vi "Perform Search Packages.vi"(9 "Filters":T1, 10 "SearchCriteria":string, 11 "All Packages":refnum<class "Package.lvclass">[](array[class])) -> (3 "Found Packages":refnum<class "Package.lvclass">[](array[class]))   [LabVIEW 2020, in "WSsupport.lvlib"]
uses:
  WSsupport.lvlib
  Packages/Package_class/Package.lvclass
  Packages/Package Version_class/Package Version.lvclass
  Search Filters.ctl
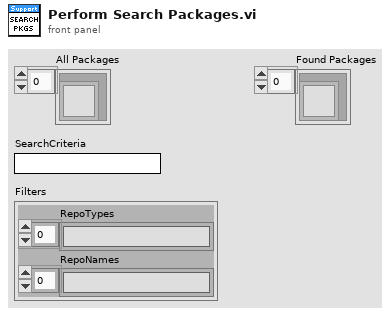
[diagram p1: front panel]
types:
  T1 = typedef "WSsupport.lvlib/Search Filters.ctl" = cluster{"RepoTypes":string[], "RepoNames":string[]}
  T2 = typedef "Packages.lvlib/Repo.lvclass/RepoType--enum.ctl" = enum16{"VIPM", "NIPM", "GPM"}
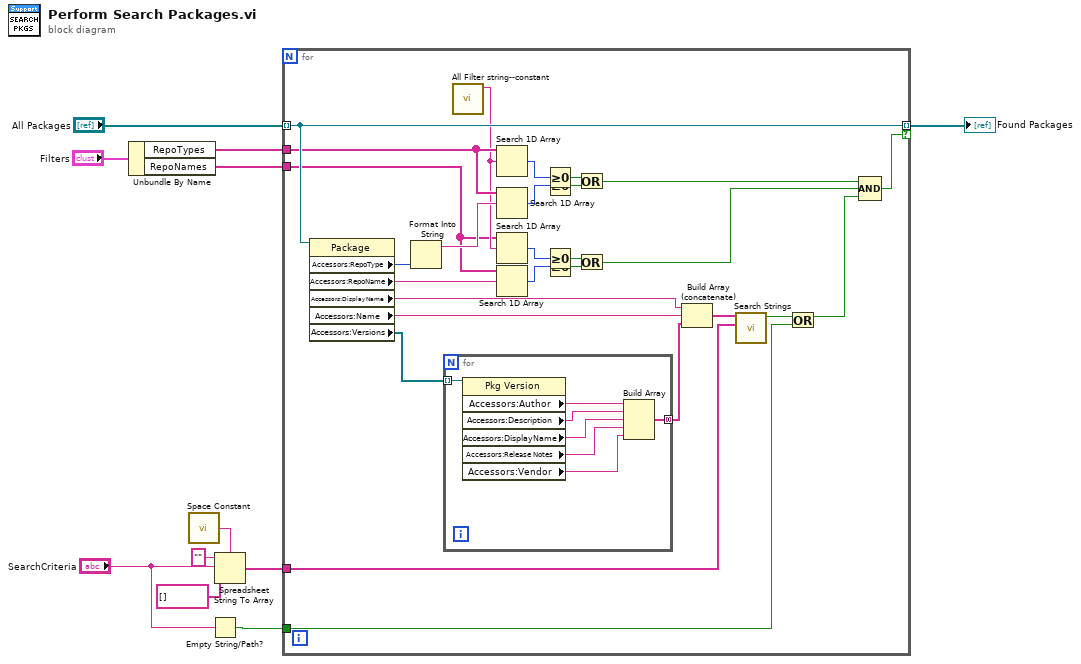
[diagram p0: block diagram]
diagram:
  n1 = Unbundle By Name("Filters") -> ("RepoTypes"=w2:string[], "RepoNames"=w1:string[])
  n2 = call <vilib>:"Space Constant.vi"() -> ("String"=w7:string)
  n3 = Empty String/Path?(string/path="SearchCriteria") -> (empty?=w4:bool)
  n4 = Spreadsheet String To Array(delimiter (Tab)=w7, format string="", spreadsheet string="SearchCriteria", array type (2D Dbl)=string[] []) -> (array=w5:string[])
  n5 = for {
    tunnel: "All Packages" -> [w37] mode=indexing
    tunnel: w5 -> [w32]
    tunnel: [w37] -> w10 mode=indexing if=w27
    tunnel: w4 -> [w29]
    tunnel: w2 -> [w26]
    tunnel: w1 -> [w19]
    n6 = property class="Package"(reference=w37) -> ("Accessors:RepoType"=w28:T2, "Accessors:RepoName"=w20:string, "Accessors:DisplayName"=w35:string, "Accessors:Name"=w34:string, "Accessors:Versions"=w38:refnum<class "Package Version.lvclass">[])  [unwired: 1 in, 2 out]
    n7 = Format Into String(w28) -> (resulting string=w25:string)  [unwired: 3 in, 1 out]
    n8 = for {
      tunnel: w38 -> [w45] mode=indexing
      tunnel: [w39] -> w36 mode=concatenating
      n9 = property class="Pkg Version"(reference=w45) -> ("Accessors:Author"=w44:string, "Accessors:Description"=w43:string, "Accessors:DisplayName"=w42:string, "Accessors:Release Notes"=w41:string, "Accessors:Vendor"=w40:string)  [unwired: 1 in, 2 out]
      n10 = Build Array(w44, w43, w42, w41, w40) -> (w39:string[])
    }
    n11 = call "All Filter string--constant.vi"() -> ("All Filter string"=w21:string)  [unwired: 11 in]
    n12 = Search 1D Array(1D array=w26, element=w21) -> (index of element=w24:i32)  [unwired: 1 in]
    n13 = Search 1D Array(1D array=w26, element=w25) -> (index of element=w23:i32)  [unwired: 1 in]
    n14 = Search 1D Array(1D array=w19, element=w21) -> (index of element=w14:i32)  [unwired: 1 in]
    n15 = Search 1D Array(1D array=w19, element=w20) -> (index of element=w13:i32)  [unwired: 1 in]
    n16 = Greater Or Equal To 0?(x=w24) -> (x >= 0?=w18:bool)
    n17 = Greater Or Equal To 0?(x=w23) -> (x >= 0?=w17:bool)
    n18 = Greater Or Equal To 0?(x=w14) -> (x >= 0?=w15:bool)
    n19 = Greater Or Equal To 0?(x=w13) -> (x >= 0?=w16:bool)
    n20 = Or(x=w18, y=w17) -> (x .or. y?=w22:bool)
    n21 = Or(x=w15, y=w16) -> (x .or. y?=w12:bool)
    n22 = Build Array (concatenate)(w35, w34, w36) -> (w33:string[])
    n23 = call "Search Strings.vi"("Search Strings"=w32, "Strings to be looked"=w33) -> ("Found?"=w31:bool)  [unwired: 9 in]
    n24 = Or(x=w31, y=w29) -> (x .or. y?=w30:bool)
    n25 = Compound Arithmetic op=AND(w22, w12, w30) -> (w27:bool)
  }
  "Found Packages" <- w10
